vi "IR_Sensor_Movement_and_Math.vi"(11 "Position 1":u8) -> (0 "Minimum":i16, 3 "Maximum":i16)   [LabVIEW 2012, in "Serenity_mk2.lvrbt"]
uses:
  Serenity_mk2.lvrbt
  <vilib>/NXT/Hardware/Plugins/Tetrix 180 deg Servo/Tetrix180ServoAddress.ctl
  <vilib>/NXT/HiTechnic/HiTechnic Controls/HiTechnic Port.ctl
  <vilib>/NXT/Block Support/NXT_InputPort.ctl
  <vilib>/NXT/NXTIO Xnodes/NXTIONodeSubVIs/TETRIX IO Move Servos.vi
  <vilib>/NXT/Dual Mode Library/prims/inRangeAndCoerce/inRangeAndCoerce_float.vi
  <vilib>/NXT/Subs/LVHSConnector.ctl
  <vilib>/NXT/NXTIO Xnodes/AddressXNode/NXTIOAddress.xnode
  <vilib>/NXT/NXTIO Xnodes/NXTIOXNode/NXTIO.xnode
  <vilib>/NXT/LegoClasses/BrickReference/BrickReference.lvclass
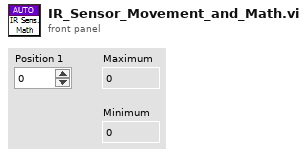
[diagram p1: front panel]
types:
  T1 = typedef "HiTechnic Port.ctl" = cluster{"Port":T2, "MUX Port":u8}
  T2 = typedef "NXT_InputPort.ctl" = u32
  T3 = typedef "Tetrix180ServoAddress.ctl" = i32
  T4 = cluster{"Direction (0-9)":i16, "Signal Strength (Array)":u8[]}
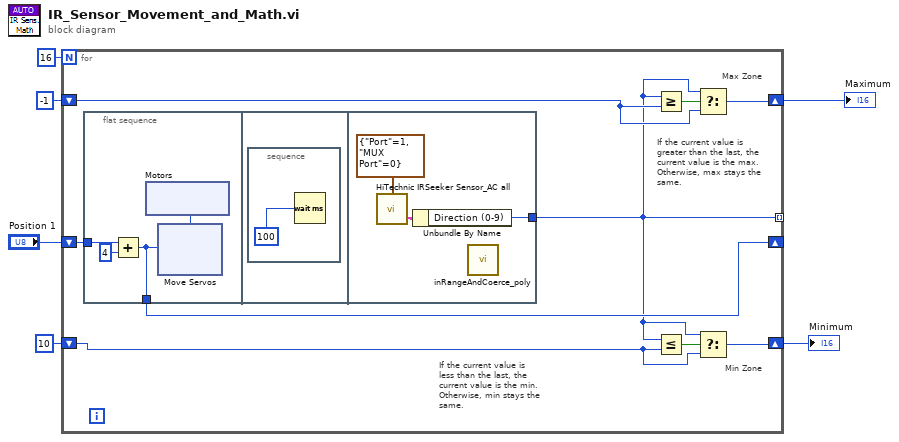
[diagram p0: block diagram]
diagram:
  n1 = for {
    N: 16 -> [_]
    tunnel: [w7] -> _ mode=indexing
    shift-right: [w9] -> _
    shift-left: "Position 1" -> [w15]
    shift-right: [w13] -> w6
    shift-left: i16 -1 ("Direction (0-9)") -> [w12]
    shift-right: [w10] -> w5
    shift-left: i16 10 ("Direction (0-9)") -> [w8]
    # "If the current value is\nless than the last, the\ncurrent value is the min.\nOtherwise, min stays the\nsame."
    # "If the current value is\ngreater than the last, the\ncurrent value is the max.\nOtherwise, max stays the\nsame."
    # "Min Zone"
    # "Max Zone"
    n2 = flat-sequence {
      tunnel: w15 -> [w17]
      tunnel: [w16] -> w9
      tunnel: [w29] -> w7
      frame #0 {
        n3 = Add(x=w17, y=u8 4) -> (x+y=w16:u8)
        n4 = xnode "Motors"() -> ("Motor"=w19:T3)
        n5 = xnode "Move Servos"("Position 1"=w16, "Motors"=w19) -> ()  [unwired: 1 in, 1 out]
      }
      frame #1 {
        n6 = stacked-sequence {
          frame #0 {
            n7 = Wait (ms)(milliseconds to wait=u32 100 ("Time (1 sec)")) -> ()  [unwired: 1 out]
          }
        }
      }
      frame #2 {
        n8 = call <vilib>:"HiTechnic IRSeeker Sensor_AC all.vi"("Port/MUX"=T1 {"Port"=1, "MUX Port"=0}) -> ("All Info"=w31:T4)  [unwired: 2 in, 1 out]
        n9 = Unbundle By Name(w31) -> ("Direction (0-9)"=w29:i16)
        n10 = call-poly <vilib>:"inRangeAndCoerce_poly.vi"() -> ()  [unwired: 3 in, 2 out]
      }
    }
    n11 = Greater Or Equal?(x=w7, y=w12) -> (x >= y?=w14:bool)
    n12 = Less Or Equal?(x=w7, y=w8) -> (x <= y?=w11:bool)
    n13 = Select(t=w7, s=w14, f=w12) -> (s? t:f=w13:i16)
    n14 = Select(t=w7, s=w11, f=w8) -> (s? t:f=w10:i16)
  }
  "Maximum" <- w6
  "Minimum" <- w5
